vi "TIO Format Stream.vi"(7 "Type(T:GMR)":bool, 8 "entrée d'erreur (pas d'erreur)":errorcluster, 9 "TIO State":T2={"Awaiting REP"=FALSE, "REQ ID"=500, "dstreams in"=[{"id"=0, "timebase id"=1, "period"=4, "offset"=0, "sample number"=914806, "total components"=5, "flags"=1, "components"=[{"pstream id"=0, "flags"=0, "period"=1, "offset"=0}, {"pstream id"=1, "flags"=1, "period"=5, "offset"=0}, {"pstream id"=2, "flags"=1, "period"=5, "offset"=0}, {"pstream id"=3, "flags"=0, "period"=100, "offset"=0}, {"pstream id"=4, "flags"=0, "period"=100, "offset"=0}]}, {"id"=0, "timebase id"=0, "period"=0, "offset"=0, "sample number"=0, "total components"=0, "flags"=0, "components"=[]}, {"id"=0, "timebase id"=0, "period"=0, "offset"=0, "sample number"=0, "total components"=0, "flags"=0, "components"=[]}, {"id"=0, "timebase id"=0, "period"=0, "offset"=0, "sample number"=0, "total components"=0, "flags"=0, "components"=[]}, {"id"=0, "timebase id"=0, "period"=0, "offset"=0, "sample number"=0, "total components"=0, "flags"=0, "components"=[]}, {"id"=0, "timebase id"=0, "period"=0, "offset"=0, "sample number"=0, "total components"=0, "flags"=0, "components"=[]}, {"id"=0, "timebase id"=0, "period"=0, "offset"=0, "sample number"=0, "total components"=0, "flags"=0, "components"=[]}, {"id"=0, "timebase id"=0, "period"=0, "offset"=0, "sample number"=0, "total components"=0, "flags"=0, "components"=[]}, {"id"=0, "timebase id"=0, "period"=0, "offset"=0, "sample number"=0, "total components"=0, "flags"=0, "components"=[]}, {"id"=0, "timebase id"=0, "period"=0, "offset"=0, "sample number"=0, "total components"=0, "flags"=0, "components"=[]}, {"id"=0, "timebase id"=0, "period"=0, "offset"=0, "sample number"=0, "total components"=0, "flags"=0, "components"=[]}, {"id"=0, "timebase id"=0, "period"=0, "offset"=0, "sample number"=0, "total components"=0, "flags"=0, "components"=[]}, {"id"=0, "timebase id"=0, "period"=0, "offset"=0, "sample number"=0, "total components"=0, "flags"=0, "components"=[]}, {"id"=0, "timebase id"=0, "period"=0, "offset"=0, "sample number"=0, "total components"=0, "flags"=0, "components"=[]}, {"id"=0, "timebase id"=0, "period"=0, "offset"=0, "sample number"=0, "total components"=0, "flags"=0, "components"=[]}, {"id"=0, "timebase id"=0, "period"=0, "offset"=0, "sample number"=0, "total components"=0, "flags"=0, "components"=[]}, {"id"=0, "timebase id"=0, "period"=0, "offset"=0, "sample number"=0, "total components"=0, "flags"=0, "components"=[]}, {"id"=0, "timebase id"=0, "period"=0, "offset"=0, "sample number"=0, "total components"=0, "flags"=0, "components"=[]}, {"id"=0, "timebase id"=0, "period"=0, "offset"=0, "sample number"=0, "total components"=0, "flags"=0, "components"=[]}, {"id"=0, "timebase id"=0, "period"=0, "offset"=0, "sample number"=0, "total components"=0, "flags"=0, "components"=[]}, {"id"=0, "timebase id"=0, "period"=0, "offset"=0, "sample number"=0, "total components"=0, "flags"=0, "components"=[]}, {"id"=0, "timebase id"=0, "period"=0, "offset"=0, "sample number"=0, "total components"=0, "flags"=0, "components"=[]}, {"id"=0, "timebase id"=0, "period"=0, "offset"=0, "sample number"=0, "total components"=0, "flags"=0, "components"=[]}, {"id"=0, "timebase id"=0, "period"=0, "offset"=0, "sample number"=0, "total components"=0, "flags"=0, "components"=[]}, {"id"=0, "timebase id"=0, "period"=0, "offset"=0, "sample number"=0, "total components"=0, "flags"=0, "components"=[]}, {"id"=0, "timebase id"=0, "period"=0, "offset"=0, "sample number"=0, "total components"=0, "flags"=0, "components"=[]}, {"id"=0, "timebase id"=0, "period"=0, "offset"=0, "sample number"=0, "total components"=0, "flags"=0, "components"=[]}, {"id"=0, "timebase id"=0, "period"=0, "offset"=0, "sample number"=0, "total components"=0, "flags"=0, "components"=[]}, {"id"=0, "timebase id"=0, "period"=0, "offset"=0, "sample number"=0, "total components"=0, "flags"=0, "components"=[]}, {"id"=0, "timebase id"=0, "period"=0, "offset"=0, "sample number"=0, "total components"=0, "flags"=0, "components"=[]}, {"id"=0, "timebase id"=0, "period"=0, "offset"=0, "sample number"=0, "total components"=0, "flags"=0, "components"=[]}, {"id"=0, "timebase id"=0, "period"=0, "offset"=0, "sample number"=0, "total components"=0, "flags"=0, "components"=[]}], "pstreams"=[{"id"=0, "timebase_id"=1, "period"=1, "offset"=0, "fmt"=-1, "flags"=0, "channels"=3, "type"=66, "name"="gmr", "column names"=["x", "y", "z"], "title"="Vector magnetic field", "units"="nT"}, {"id"=1, "timebase_id"=1, "period"=8, "offset"=0, "fmt"=-1, "flags"=0, "channels"=3, "type"=66, "name"="accel", "column names"=["x", "y", "z"], "title"="Acceleration", "units"="m/s^2"}, {"id"=2, "timebase_id"=1, "period"=8, "offset"=0, "fmt"=-1, "flags"=0, "channels"=3, "type"=66, "name"="gyro", "column names"=["x", "y", "z"], "title"="Angular velocity", "units"="rad/s"}, {"id"=3, "timebase_id"=1, "period"=80, "offset"=0, "fmt"=-1, "flags"=0, "channels"=1, "type"=66, "name"="bar", "column names"=[""], "title"="Atmospheric pressure", "units"="mbar"}, {"id"=4, "timebase_id"=1, "period"=80, "offset"=0, "fmt"=-1, "flags"=0, "channels"=1, "type"=66, "name"="therm", "column names"=[""], "title"="Ambient temperature", "units"="C"}, {"id"=0, "timebase_id"=0, "period"=0, "offset"=0, "fmt"=0, "flags"=0, "channels"=0, "type"=0, "name"="", "column names"=[], "title"="", "units"=""}, {"id"=0, "timebase_id"=0, "period"=0, "offset"=0, "fmt"=0, "flags"=0, "channels"=0, "type"=0, "name"="", "column names"=[], "title"="", "units"=""}, {"id"=0, "timebase_id"=0, "period"=0, "offset"=0, "fmt"=0, "flags"=0, "channels"=0, "type"=0, "name"="", "column names"=[], "title"="", "units"=""}, {"id"=0, "timebase_id"=0, "period"=0, "offset"=0, "fmt"=0, "flags"=0, "channels"=0, "type"=0, "name"="", "column names"=[], "title"="", "units"=""}, {"id"=0, "timebase_id"=0, "period"=0, "offset"=0, "fmt"=0, "flags"=0, "channels"=0, "type"=0, "name"="", "column names"=[], "title"="", "units"=""}, {"id"=0, "timebase_id"=0, "period"=0, "offset"=0, "fmt"=0, "flags"=0, "channels"=0, "type"=0, "name"="", "column names"=[], "title"="", "units"=""}, {"id"=0, "timebase_id"=0, "period"=0, "offset"=0, "fmt"=0, "flags"=0, "channels"=0, "type"=0, "name"="", "column names"=[], "title"="", "units"=""}, {"id"=0, "timebase_id"=0, "period"=0, "offset"=0, "fmt"=0, "flags"=0, "channels"=0, "type"=0, "name"="", "column names"=[], "title"="", "units"=""}, {"id"=0, "timebase_id"=0, "period"=0, "offset"=0, "fmt"=0, "flags"=0, "channels"=0, "type"=0, "name"="", "column names"=[], "title"="", "units"=""}, {"id"=0, "timebase_id"=0, "period"=0, "offset"=0, "fmt"=0, "flags"=0, "channels"=0, "type"=0, "name"="", "column names"=[], "title"="", "units"=""}, {"id"=0, "timebase_id"=0, "period"=0, "offset"=0, "fmt"=0, "flags"=0, "channels"=0, "type"=0, "name"="", "column names"=[], "title"="", "units"=""}, {"id"=32768, "timebase_id"=1, "period"=1, "offset"=0, "fmt"=-1, "flags"=0, "channels"=3, "type"=66, "name"="_gmr.raw", "column names"=["x", "y", "z"], "title"="Vector magnetic field", "units"="nT"}, {"id"=32769, "timebase_id"=1, "period"=8, "offset"=0, "fmt"=-1, "flags"=0, "channels"=3, "type"=66, "name"="_accel.raw", "column names"=["x", "y", "z"], "title"="Acceleration", "units"="m/s^2"}, {"id"=32770, "timebase_id"=1, "period"=8, "offset"=0, "fmt"=-1, "flags"=0, "channels"=3, "type"=66, "name"="_gyro.raw", "column names"=["x", "y", "z"], "title"="Angular velocity", "units"="rad/s"}, {"id"=32771, "timebase_id"=1, "period"=80, "offset"=0, "fmt"=-1, "flags"=0, "channels"=1, "type"=66, "name"="_bar.raw", "column names"=[""], "title"="Atmospheric pressure", "units"="mbar"}, {"id"=32772, "timebase_id"=1, "period"=80, "offset"=0, "fmt"=-1, "flags"=0, "channels"=1, "type"=66, "name"="_therm.raw", "column names"=[""], "title"="Ambient temperature", "units"="C"}, {"id"=32773, "timebase_id"=0, "period"=1, "offset"=0, "fmt"=-1, "flags"=0, "channels"=1, "type"=66, "name"="_cpu.raw", "column names"=[""], "title"="CPU load", "units"="%"}, {"id"=32774, "timebase_id"=0, "period"=1, "offset"=0, "fmt"=-1, "flags"=0, "channels"=1, "type"=66, "name"="cpu", "column names"=[""], "title"="CPU load", "units"="%"}, {"id"=0, "timebase_id"=0, "period"=0, "offset"=0, "fmt"=0, "flags"=0, "channels"=0, "type"=0, "name"="", "column names"=[], "title"="", "units"=""}, {"id"=0, "timebase_id"=0, "period"=0, "offset"=0, "fmt"=0, "flags"=0, "channels"=0, "type"=0, "name"="", "column names"=[], "title"="", "units"=""}, {"id"=0, "timebase_id"=0, "period"=0, "offset"=0, "fmt"=0, "flags"=0, "channels"=0, "type"=0, "name"="", "column names"=[], "title"="", "units"=""}, {"id"=0, "timebase_id"=0, "period"=0, "offset"=0, "fmt"=0, "flags"=0, "channels"=0, "type"=0, "name"="", "column names"=[], "title"="", "units"=""}, {"id"=0, "timebase_id"=0, "period"=0, "offset"=0, "fmt"=0, "flags"=0, "channels"=0, "type"=0, "name"="", "column names"=[], "title"="", "units"=""}, {"id"=0, "timebase_id"=0, "period"=0, "offset"=0, "fmt"=0, "flags"=0, "channels"=0, "type"=0, "name"="", "column names"=[], "title"="", "units"=""}, {"id"=0, "timebase_id"=0, "period"=0, "offset"=0, "fmt"=0, "flags"=0, "channels"=0, "type"=0, "name"="", "column names"=[], "title"="", "units"=""}, {"id"=0, "timebase_id"=0, "period"=0, "offset"=0, "fmt"=0, "flags"=0, "channels"=0, "type"=0, "name"="", "column names"=[], "title"="", "units"=""}, {"id"=0, "timebase_id"=0, "period"=0, "offset"=0, "fmt"=0, "flags"=0, "channels"=0, "type"=0, "name"="", "column names"=[], "title"="", "units"=""}], "timebases"=[{"id"=0, "source"=513, "epoch"=0, "start time"=0, "period numerator (µs)"=100000000, "period denominator (µs)"=1000, "flags"=0, "stability"=1, "source id"="\u0000\u0000\u0000¬Å'7\u0001\u0000\u0000\u0000B\u0000!\u0000\u0011P6W462 "}, {"id"=1, "source"=513, "epoch"=194250488, "start time"=0, "period numerator (µs)"=1250000, "period denominator (µs)"=1000, "flags"=0, "stability"=1, "source id"="\u0000\u0000\u0000¬Å'7\u0001\u0000\u0000\u0000B\u0000!\u0000\u0011P6W462 "}, {"id"=0, "source"=0, "epoch"=0, "start time"=0, "period numerator (µs)"=0, "period denominator (µs)"=0, "flags"=0, "stability"=0, "source id"=""}, {"id"=0, "source"=0, "epoch"=0, "start time"=0, "period numerator (µs)"=0, "period denominator (µs)"=0, "flags"=0, "stability"=0, "source id"=""}, {"id"=0, "source"=0, "epoch"=0, "start time"=0, "period numerator (µs)"=0, "period denominator (µs)"=0, "flags"=0, "stability"=0, "source id"=""}, {"id"=0, "source"=0, "epoch"=0, "start time"=0, "period numerator (µs)"=0, "period denominator (µs)"=0, "flags"=0, "stability"=0, "source id"=""}, {"id"=0, "source"=0, "epoch"=0, "start time"=0, "period numerator (µs)"=0, "period denominator (µs)"=0, "flags"=0, "stability"=0, "source id"=""}, {"id"=0, "source"=0, "epoch"=0, "start time"=0, "period numerator (µs)"=0, "period denominator (µs)"=0, "flags"=0, "stability"=0, "source id"=""}, {"id"=0, "source"=0, "epoch"=0, "start time"=0, "period numerator (µs)"=0, "period denominator (µs)"=0, "flags"=0, "stability"=0, "source id"=""}, {"id"=0, "source"=0, "epoch"=0, "start time"=0, "period numerator (µs)"=0, "period denominator (µs)"=0, "flags"=0, "stability"=0, "source id"=""}, {"id"=0, "source"=0, "epoch"=0, "start time"=0, "period numerator (µs)"=0, "period denominator (µs)"=0, "flags"=0, "stability"=0, "source id"=""}, {"id"=0, "source"=0, "epoch"=0, "start time"=0, "period numerator (µs)"=0, "period denominator (µs)"=0, "flags"=0, "stability"=0, "source id"=""}, {"id"=0, "source"=0, "epoch"=0, "start time"=0, "period numerator (µs)"=0, "period denominator (µs)"=0, "flags"=0, "stability"=0, "source id"=""}, {"id"=0, "source"=0, "epoch"=0, "start time"=0, "period numerator (µs)"=0, "period denominator (µs)"=0, "flags"=0, "stability"=0, "source id"=""}, {"id"=0, "source"=0, "epoch"=0, "start time"=0, "period numerator (µs)"=0, "period denominator (µs)"=0, "flags"=0, "stability"=0, "source id"=""}, {"id"=0, "source"=0, "epoch"=0, "start time"=0, "period numerator (µs)"=0, "period denominator (µs)"=0, "flags"=0, "stability"=0, "source id"=""}, {"id"=0, "source"=0, "epoch"=0, "start time"=0, "period numerator (µs)"=0, "period denominator (µs)"=0, "flags"=0, "stability"=0, "source id"=""}, {"id"=0, "source"=0, "epoch"=0, "start time"=0, "period numerator (µs)"=0, "period denominator (µs)"=0, "flags"=0, "stability"=0, "source id"=""}, {"id"=0, "source"=0, "epoch"=0, "start time"=0, "period numerator (µs)"=0, "period denominator (µs)"=0, "flags"=0, "stability"=0, "source id"=""}, {"id"=0, "source"=0, "epoch"=0, "start time"=0, "period numerator (µs)"=0, "period denominator (µs)"=0, "flags"=0, "stability"=0, "source id"=""}, {"id"=0, "source"=0, "epoch"=0, "start time"=0, "period numerator (µs)"=0, "period denominator (µs)"=0, "flags"=0, "stability"=0, "source id"=""}, {"id"=0, "source"=0, "epoch"=0, "start time"=0, "period numerator (µs)"=0, "period denominator (µs)"=0, "flags"=0, "stability"=0, "source id"=""}, {"id"=0, "source"=0, "epoch"=0, "start time"=0, "period numerator (µs)"=0, "period denominator (µs)"=0, "flags"=0, "stability"=0, "source id"=""}, {"id"=0, "source"=0, "epoch"=0, "start time"=0, "period numerator (µs)"=0, "period denominator (µs)"=0, "flags"=0, "stability"=0, "source id"=""}, {"id"=0, "source"=0, "epoch"=0, "start time"=0, "period numerator (µs)"=0, "period denominator (µs)"=0, "flags"=0, "stability"=0, "source id"=""}, {"id"=0, "source"=0, "epoch"=0, "start time"=0, "period numerator (µs)"=0, "period denominator (µs)"=0, "flags"=0, "stability"=0, "source id"=""}, {"id"=0, "source"=0, "epoch"=0, "start time"=0, "period numerator (µs)"=0, "period denominator (µs)"=0, "flags"=0, "stability"=0, "source id"=""}, {"id"=0, "source"=0, "epoch"=0, "start time"=0, "period numerator (µs)"=0, "period denominator (µs)"=0, "flags"=0, "stability"=0, "source id"=""}, {"id"=0, "source"=0, "epoch"=0, "start time"=0, "period numerator (µs)"=0, "period denominator (µs)"=0, "flags"=0, "stability"=0, "source id"=""}, {"id"=0, "source"=0, "epoch"=0, "start time"=0, "period numerator (µs)"=0, "period denominator (µs)"=0, "flags"=0, "stability"=0, "source id"=""}, {"id"=0, "source"=0, "epoch"=0, "start time"=0, "period numerator (µs)"=0, "period denominator (µs)"=0, "flags"=0, "stability"=0, "source id"=""}, {"id"=0, "source"=0, "epoch"=0, "start time"=0, "period numerator (µs)"=0, "period denominator (µs)"=0, "flags"=0, "stability"=0, "source id"=""}]}, 10 "Payload":string, 11 "Packet Type":u16) -> (0 "sortie d'erreur":errorcluster, 1 "dstream info":T3, 2 "pstreams out":T4(array[cluster]), 3 "Data Out":T1(array[cluster])=[{"Name"="gmr", "Waveform"={"start"=0.0, "dt"=1.0, "Timeseries"=[[-1045203.625, 2103369.25, -524451.0625]]}}, {"Name"="accel", "Waveform"={"start"=0.0, "dt"=1.0, "Timeseries"=[[0.4673272967338562, -9.214466094970703, -3.09728741645813]]}}, {"Name"="gyro", "Waveform"={"start"=0.0, "dt"=1.0, "Timeseries"=[[0.019417261704802513, 0.00881516095250845, 0.006293708924204111]]}}, {"Name"="bar", "Waveform"={"start"=0.0, "dt"=1.0, "Timeseries"=[[0.0]]}}, {"Name"="therm", "Waveform"={"start"=0.0, "dt"=1.0, "Timeseries"=[[0.0]]}}] {"Waveform"."start" format="%#.3f"}, 4 "timebases out":T5(array[cluster]))   [LabVIEW 2010]
panel:
  out "Sample number":u32
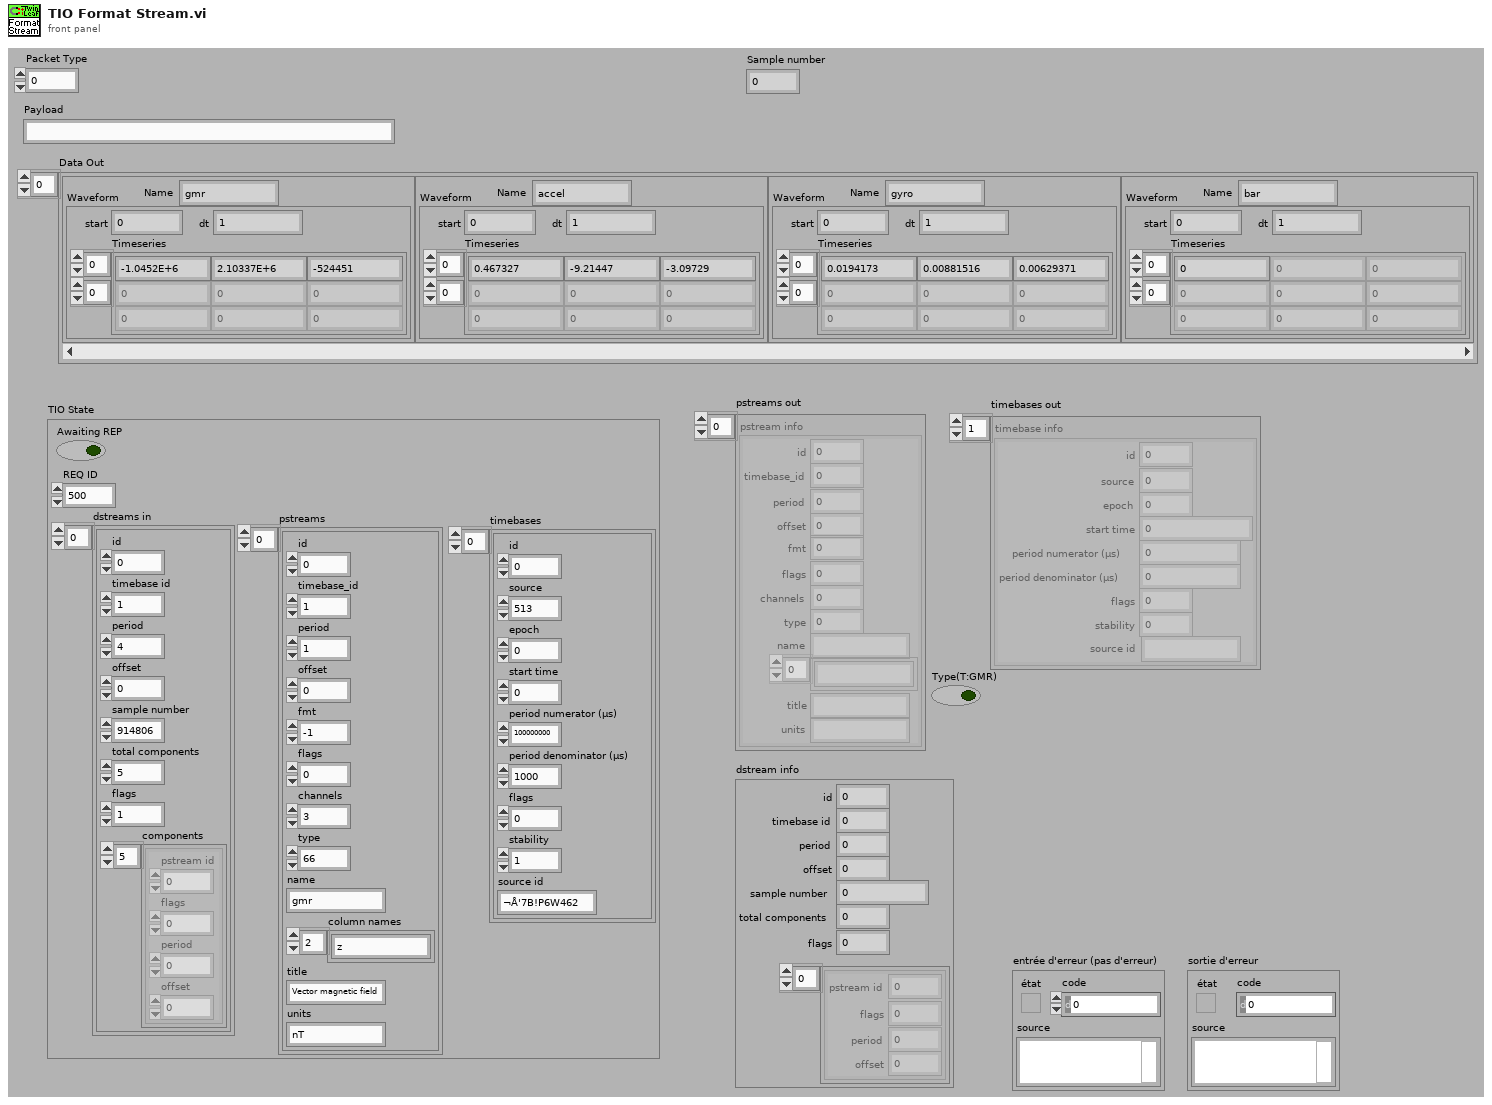
[diagram p1: front panel]
types:
  T1 = cluster{"Name":string, "Waveform":cluster{"start":dbl, "dt":dbl, "Timeseries":dbl[][]}}[]
  T2 = cluster{"Awaiting REP":bool, "REQ ID":u32, "dstreams in":cluster{"id":u16, "timebase id":u16, "period":u32, "offset":u32, "sample number":u64, "total components":u16, "flags":u16, "components":cluster{"pstream id":u16, "flags":u16, "period":u32, "offset":u32}[]}[], "pstreams":cluster{"id":u16, "timebase_id":u16, "period":u32, "offset":u32, "fmt":i32, "flags":u16, "channels":u16, "type":u8, "name":string, "column names":string[], "title":string, "units":string}[], "timebases":cluster{"id":u16, "source":u16, "epoch":u32, "start time":u32, "period numerator (µs)":i32, "period denominator (µs)":u16, "flags":u16, "stability":u8, "source id":string}[]}
  T3 = cluster{"id":u16, "timebase id":u16, "period":u32, "offset":u32, "sample number":u64, "total components":u16, "flags":u16, cluster{"pstream id":u16, "flags":u16, "period":u32, "offset":u32}[]}
  T4 = cluster{"id":u16, "timebase_id":u16, "period":u32, "offset":u32, "fmt":i32, "flags":u16, "channels":u16, "type":u8, "name":string, string[], "title":string, "units":string}[]
  T5 = cluster{"id":u16, "source":u8, "epoch":u8, "start time":u64, "period numerator (µs)":u32, "period denominator (µs)":u32, "flags":u32, "stability":sgl, "source id":string}[]
  T6 = enum16{"big-endian, network order", "native, host order", "little-endian"}
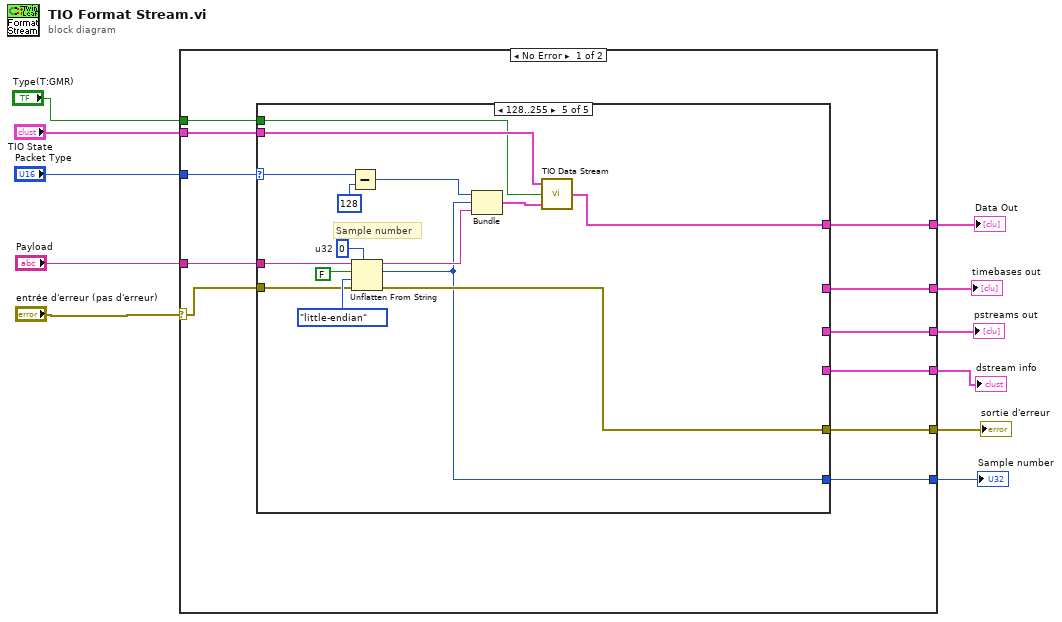
[diagram p0: block diagram]
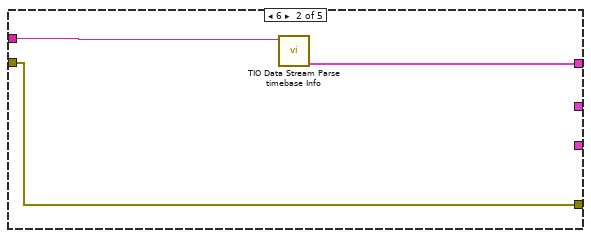
[diagram p3: hidden frame]
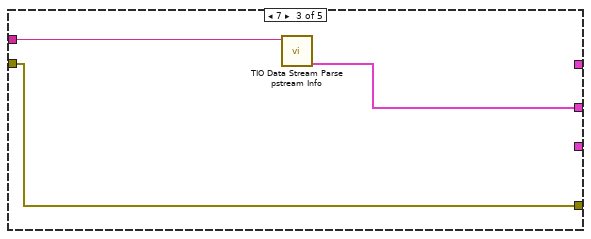
[diagram p4: hidden frame]
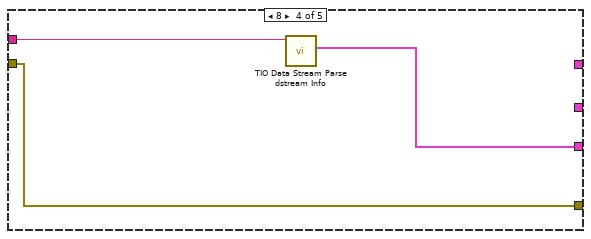
[diagram p5: hidden frame]
diagram:
  n1 = case shown="No Error" "entrée d'erreur (pas d'erreur)" {
    selector: "entrée d'erreur (pas d'erreur)" -> [w19 w48]
    tunnel: "Payload" -> [w22 _]
    tunnel: "Packet Type" -> [w21 _]
    tunnel: "TIO State" -> [w20 _]
    tunnel: [w18 _] -> w7
    tunnel: [w17 _] -> w6
    tunnel: [w16 _] -> w5
    tunnel: [w15 _] -> w4
    tunnel: [w14 w48] -> w3
    tunnel: [w13 _] -> w2
    tunnel: "Type(T:GMR)" -> [w12 _]
    frame No Error {
      n2 = case shown="128..255" w21 {
        selector: w21 -> [_ _ _ _ w41]
        tunnel: w22 -> [_ w26 w29 w32 w40]
        tunnel: w20 -> [_ _ _ _ w38]
        tunnel: w19 -> [w23 w24 w27 w30 w37]
        tunnel: [_ w25 _ _ _] -> w18
        tunnel: [_ _ w28 _ _] -> w17
        tunnel: [_ _ _ w31 _] -> w16
        tunnel: [_ _ _ _ w36] -> w15
        tunnel: [w23 w24 w27 w30 w35] -> w14
        tunnel: [_ _ _ _ w34] -> w13
        tunnel: w12 -> [_ _ _ _ w33]
        frame Default {
        }
        frame 6 {
          n3 = call <userlib>:"TIO Data Stream Parse timebase Info.vi"("timebase info raw"=w26) -> ("timebases out"=w25:T5)  [unwired: 10 in]
        }
        frame 7 {
          n4 = call <userlib>:"TIO Data Stream Parse pstream Info.vi"("pstream info raw"=w29) -> ("pstreams out"=w28:T4)  [unwired: 10 in]
        }
        frame 8 {
          n5 = call <userlib>:"TIO Data Stream Parse dstream Info.vi"("dstream info raw"=w32) -> ("dstream info"=w31:T3)  [unwired: 9 in, 1 out]
        }
        frame 128..255 {
          w43 = u32 0  # u32
          # "Sample number"
          n6 = Subtract(x=w41, y=u16 128) -> (x-y=w46:u16)
          n7 = Unflatten From String(type=w43, binary string=w40, data includes array or string size? (T)=FALSE, byte order (0:big-endian, network order)=T6."little-endian", error in (no error)=w37) -> (rest of the binary string=w42:string, value=w34:u32, error out=w35:errorcluster)
          n8 = Bundle(w46, "u32"=w34, w42) -> (w39:cluster{u16, "u32":u32, string})  [unwired: 1 in]
          n9 = call <userlib>:"TIO Data Stream.vi"("Raw Data"=w39, "Type(T:GMR)"=w33, "TIO State GMR"=w38) -> ("Data Out"=w36:T1)
        }
      }
    }
    frame Error {
    }
  }
  "timebases out" <- w7
  "pstreams out" <- w6
  "dstream info" <- w5
  "Data Out" <- w4
  "sortie d'erreur" <- w3
  "Sample number" <- w2
